vi "w.vi"(1 "関数":T1(ring), 2 "y":dbl, 3 "x":dbl) -> (0 "ret":dbl)   [LabVIEW 2013]
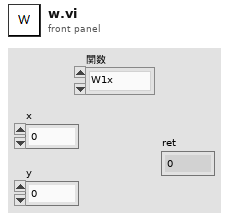
[diagram p1: front panel]
types:
  T1 = enum16{"W1x", "W1y", "W2x", "W2y", "W3x", "W3y", "W4x", "W4y"}
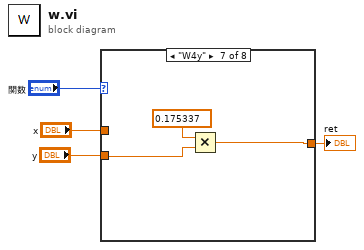
[diagram p0: block diagram]
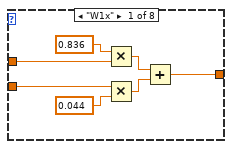
[diagram p2: hidden frame]
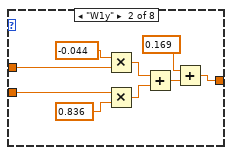
[diagram p3: hidden frame]
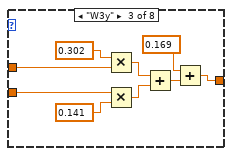
[diagram p4: hidden frame]
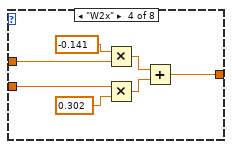
[diagram p5: hidden frame]
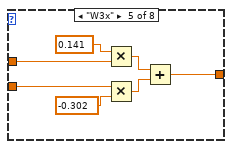
[diagram p6: hidden frame]
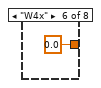
[diagram p7: hidden frame]
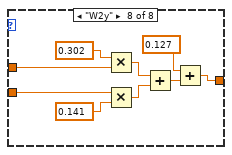
[diagram p8: hidden frame]
diagram:
  n1 = case shown="\"W4y\"" "関数" {
    tunnel: "x" -> [w10 w19 w28 w35 w42 _ _ w55]
    tunnel: "y" -> [w8 w17 w26 w33 w40 _ w47 w53]
    tunnel: [w5 w13 w22 w30 w37 0.0 w45 w49] -> w4
    frame "W1x" {
      n2 = Multiply(x=0.836, y=w10) -> (x*y=w7:dbl)
      n3 = Multiply(x=w8, y=0.044) -> (x*y=w6:dbl)
      n4 = Add(x=w7, y=w6) -> (x+y=w5:dbl)
    }
    frame "W1y" {
      n5 = Multiply(x=-0.044, y=w19) -> (x*y=w16:dbl)
      n6 = Multiply(x=w17, y=0.836) -> (x*y=w15:dbl)
      n7 = Add(x=w16, y=w15) -> (x+y=w14:dbl)
      n8 = Add(x=0.169, y=w14) -> (x+y=w13:dbl)
    }
    frame "W3y" {
      n9 = Multiply(x=0.302, y=w28) -> (x*y=w25:dbl)
      n10 = Multiply(x=w26, y=0.141) -> (x*y=w24:dbl)
      n11 = Add(x=w25, y=w24) -> (x+y=w23:dbl)
      n12 = Add(x=0.169, y=w23) -> (x+y=w22:dbl)
    }
    frame "W2x" {
      n13 = Multiply(x=-0.141, y=w35) -> (x*y=w32:dbl)
      n14 = Multiply(x=w33, y=0.302) -> (x*y=w31:dbl)
      n15 = Add(x=w32, y=w31) -> (x+y=w30:dbl)
    }
    frame "W3x" {
      n16 = Multiply(x=0.141, y=w42) -> (x*y=w39:dbl)
      n17 = Multiply(x=w40, y=-0.302) -> (x*y=w38:dbl)
      n18 = Add(x=w39, y=w38) -> (x+y=w37:dbl)
    }
    frame "W4x" {
    }
    frame "W4y" {
      n19 = Multiply(x=0.175337, y=w47) -> (x*y=w45:dbl)
    }
    frame "W2y" {
      n20 = Multiply(x=0.302, y=w55) -> (x*y=w52:dbl)
      n21 = Multiply(x=w53, y=0.141) -> (x*y=w51:dbl)
      n22 = Add(x=w52, y=w51) -> (x+y=w50:dbl)
      n23 = Add(x=0.127, y=w50) -> (x+y=w49:dbl)
    }
  }
  "ret" <- w4
